vi "JKem_Control.vi"() -> ()   [LabVIEW 2013]
uses:
  <vilib>/Instr/_visa.llb/VISA Configure Serial Port (Instr).vi
panel:
  in  "Temp Setpoint (C)":dbl
  out "Waveform Chart":cluster{dbl, dbl}(graph)
  out "Current Setpoint (C)":dbl
  in  "stop":bool
  out "error out":errorcluster
  out "Current Temp (C)":dbl
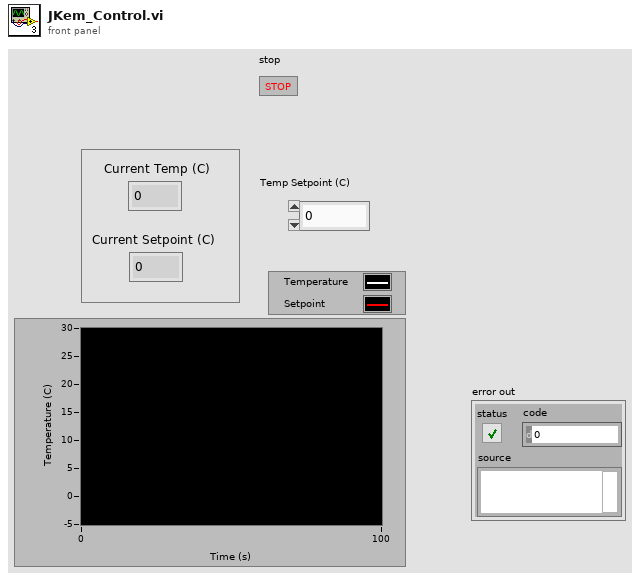
[diagram p1: front panel]
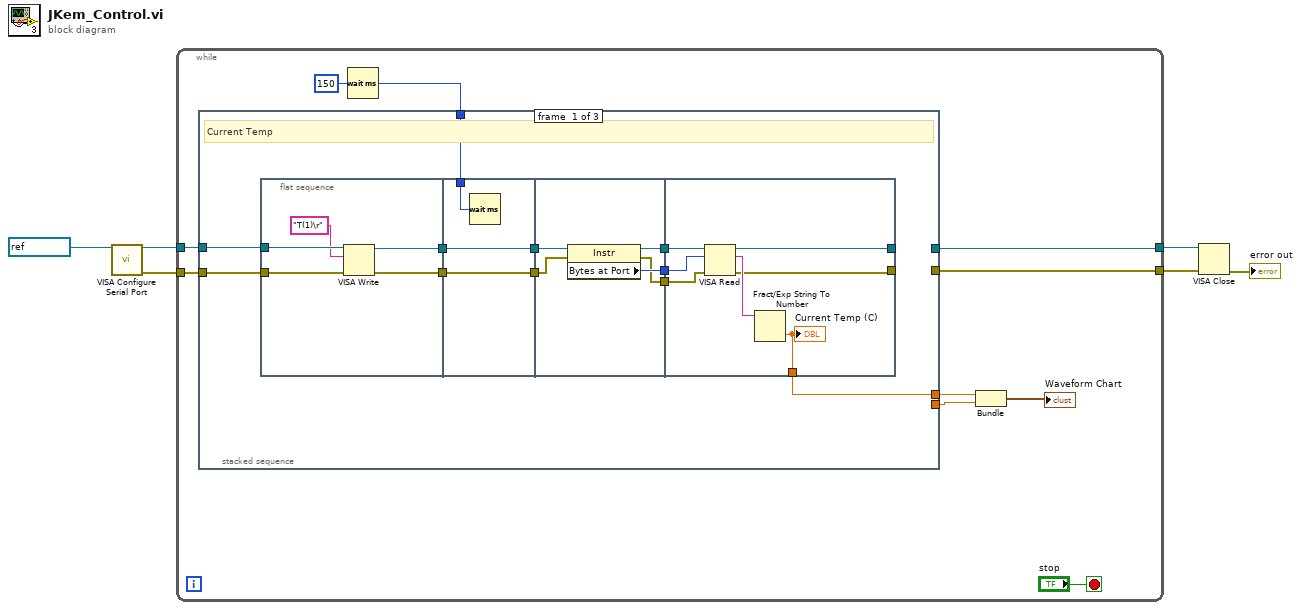
[diagram p0: block diagram]
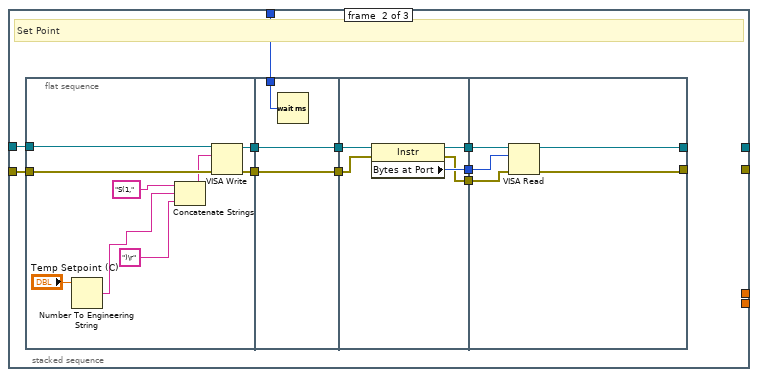
[diagram p2: hidden frame]
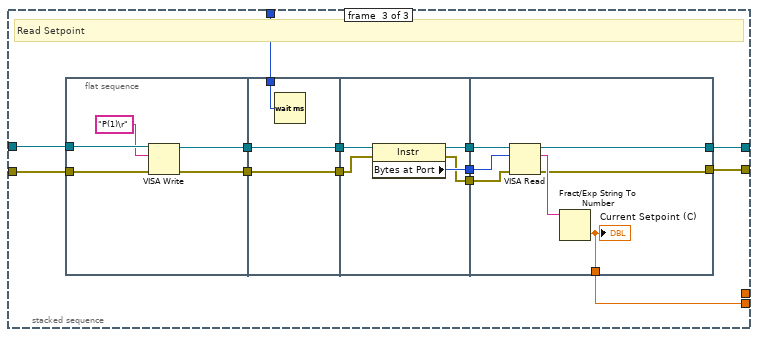
[diagram p3: hidden frame]
diagram:
  n1 = call-poly "VISA Configure Serial Port"("VISA resource name"=refnum<visa-resource-name> "COM3") -> ("VISA resource name out"=w5:refnum<visa-resource-name>, "error out"=w4:errorcluster)  [unwired: 13 in]
  n2 = while {
    tunnel: w5 -> [w15]
    tunnel: w4 -> [w14]
    tunnel: [w12] -> w3
    tunnel: [w11] -> w2
    stop <- "stop" stop-if-true
    w13 = u32 150 ("milliseconds to wait")
    n3 = stacked-sequence {
      tunnel: w15 -> [w19 w49 w83]
      tunnel: w14 -> [w18 w48 w82]
      tunnel: w13 -> [w17 w47 w84]
      tunnel: [_ _ w81] -> w12
      tunnel: [_ _ w80] -> w11
      tunnel: [w16 _ _] -> w9
      tunnel: [_ _ w79] -> w8
      frame #0 {
        # "Current Temp"
        n4 = flat-sequence {
          tunnel: w19 -> [w31]
          tunnel: w18 -> [w30]
          tunnel: [w28] -> w26
          tunnel: [w27] -> w25
          tunnel: w17 -> [w34]
          tunnel: [w33] -> w24
          tunnel: w26 -> [w33]
          tunnel: w25 -> [w32]
          tunnel: [w32] -> w23
          tunnel: w24 -> [w39]
          tunnel: w23 -> [w38]
          tunnel: [w37] -> w22
          tunnel: [w36] -> w21
          tunnel: [w35] -> w20
          tunnel: w22 -> [w46]
          tunnel: w21 -> [w45]
          tunnel: w20 -> [w44]
          tunnel: [w41] -> _
          tunnel: [w42] -> _
          tunnel: [w40] -> w16
          frame #0 {
            n5 = VISA Write(VISA resource name=w31, write buffer="T(1)\r", error in (no error)=w30) -> (VISA resource name out=w28:refnum<visa-resource-name>, error out=w27:errorcluster)  [unwired: 1 out]
          }
          frame #1 {
            n6 = Wait (ms)(milliseconds to wait=w34) -> ()  [unwired: 1 out]
          }
          frame #2 {
            n7 = property class="Instr"(reference=w39, error in=w38) -> (reference out=w37:refnum<visa-resource-name>, error out=w35:errorcluster, "Bytes at Port"=w36:u32)
          }
          frame #3 {
            n8 = VISA Read(VISA resource name=w46, byte count=w45, error in (no error)=w44) -> (VISA resource name out=w42:refnum<visa-resource-name>, read buffer=w43:string, error out=w41:errorcluster)  [unwired: 1 out]
            n9 = Fract/Exp String To Number(string=w43) -> (number=w40:dbl)  [unwired: 3 in, 1 out]
            "Current Temp (C)" <- w40
          }
        }
      }
      frame #1 {
        # "Set Point"
        n10 = flat-sequence {
          tunnel: w49 -> [w65]
          tunnel: w48 -> [w64]
          tunnel: [w63] -> w56
          tunnel: [w62] -> w55
          tunnel: w47 -> [w68]
          tunnel: [w67] -> w54
          tunnel: w56 -> [w67]
          tunnel: w55 -> [w66]
          tunnel: [w66] -> w53
          tunnel: w54 -> [w73]
          tunnel: w53 -> [w72]
          tunnel: [w71] -> w52
          tunnel: [w70] -> w51
          tunnel: [w69] -> w50
          tunnel: w52 -> [w78]
          tunnel: w51 -> [w77]
          tunnel: w50 -> [w76]
          tunnel: [w74] -> _
          tunnel: [w75] -> _
          frame #0 {
            n11 = Number To Engineering String(4:"Temp Setpoint (C)") -> (0:w58:string)  [unwired: 3 in]
            n12 = Concatenate Strings("S(1," ("write buffer"), w58, ")\r" ("write buffer")) -> (w61:string)
            n13 = VISA Write(VISA resource name=w65, write buffer=w61, error in (no error)=w64) -> (VISA resource name out=w63:refnum<visa-resource-name>, error out=w62:errorcluster)  [unwired: 1 out]
          }
          frame #1 {
            n14 = Wait (ms)(milliseconds to wait=w68) -> ()  [unwired: 1 out]
          }
          frame #2 {
            n15 = property class="Instr"(reference=w73, error in=w72) -> (reference out=w71:refnum<visa-resource-name>, error out=w69:errorcluster, "Bytes at Port"=w70:u32)
          }
          frame #3 {
            n16 = VISA Read(VISA resource name=w78, byte count=w77, error in (no error)=w76) -> (VISA resource name out=w75:refnum<visa-resource-name>, error out=w74:errorcluster)  [unwired: 2 out]
          }
        }
      }
      frame #2 {
        # "Read Setpoint"
        n17 = flat-sequence {
          tunnel: w83 -> [w96]
          tunnel: w82 -> [w95]
          tunnel: [w93] -> w91
          tunnel: [w92] -> w90
          tunnel: [w99] -> w89
          tunnel: w91 -> [w99]
          tunnel: w90 -> [w98]
          tunnel: [w98] -> w88
          tunnel: w84 -> [w97]
          tunnel: w89 -> [w104]
          tunnel: w88 -> [w103]
          tunnel: [w102] -> w87
          tunnel: [w101] -> w86
          tunnel: [w100] -> w85
          tunnel: w87 -> [w111]
          tunnel: w86 -> [w110]
          tunnel: w85 -> [w109]
          tunnel: [w106] -> w80
          tunnel: [w107] -> w81
          tunnel: [w105] -> w79
          frame #0 {
            n18 = VISA Write(VISA resource name=w96, write buffer="P(1)\r", error in (no error)=w95) -> (VISA resource name out=w93:refnum<visa-resource-name>, error out=w92:errorcluster)  [unwired: 1 out]
          }
          frame #1 {
            n19 = Wait (ms)(milliseconds to wait=w97) -> ()  [unwired: 1 out]
          }
          frame #2 {
            n20 = property class="Instr"(reference=w104, error in=w103) -> (reference out=w102:refnum<visa-resource-name>, error out=w100:errorcluster, "Bytes at Port"=w101:u32)
          }
          frame #3 {
            n21 = VISA Read(VISA resource name=w111, byte count=w110, error in (no error)=w109) -> (VISA resource name out=w107:refnum<visa-resource-name>, read buffer=w108:string, error out=w106:errorcluster)  [unwired: 1 out]
            n22 = Fract/Exp String To Number(string=w108) -> (number=w105:dbl)  [unwired: 3 in, 1 out]
            "Current Setpoint (C)" <- w105
          }
        }
      }
    }
    n23 = Wait (ms)(milliseconds to wait=w13) -> ()  [unwired: 1 out]
    n24 = Bundle(w9, w8) -> (→"Waveform Chart":cluster{dbl, dbl})  [unwired: 1 in]
  }
  n25 = VISA Close(VISA resource name=w3, error in (no error)=w2) -> (error out=→"error out":errorcluster)
